vi "Cleanup.vi"(8 "error in (no error)":errorcluster, 11 "WebProjectWatcher in":refnum<class "WebProjectWatcher.lvclass">) -> (0 "error out":errorcluster)   [LabVIEW 2020, in "PicoG-Processor.lvlib" / "WebProjectWatcher.lvclass"]
uses:
  WebProjectWatcher.lvclass
  WebProjectWatcher.lvclass/WebProjectWatcher.ctl
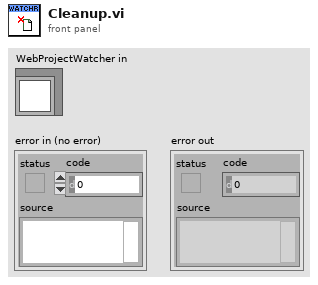
[diagram p1: front panel]
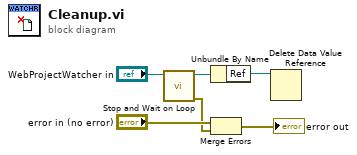
[diagram p0: block diagram]
diagram:
  n1 = call "Stop and Wait on Loop.vi"("WebProjectWatcher in"="WebProjectWatcher in") -> ("error out"=w2:errorcluster, "WebProjectWatcher out"=w4:refnum<class "WebProjectWatcher.lvclass">)  [unwired: 9 in]
  n2 = Unbundle By Name(w4) -> ("Ref"=w6:refnum<data-value>)
  n3 = Merge Errors("error in (no error)", w2) -> (→"error out":errorcluster)
  n4 = Delete Data Value Reference(data value reference=w6) -> ()  [unwired: 1 in, 2 out]
